vi "File - Load Controls from INI.vi"(7 "Section":string, 8 "error in (no error)":errorcluster, 9 "Array of References":refnum<vi>[](array[refnum]), 11 "INI File":path) -> (0 "error out":errorcluster)   [LabVIEW 2020]
doc: "Updates the values of controls (passed as an array of references) with the values read from an INI file.\n\nThe control names are used for the key names (with spaces removed).\n\nWorks with digital/boolean/string/path/VISAResourceName and single level clusters."
uses:
  <vilib>/Utility/config.llb/Read Key (Double).vi
  <vilib>/Utility/config.llb/Read Key (U32).vi
  <vilib>/Utility/config.llb/Read Key (String).vi
  <vilib>/Utility/config.llb/NI_LVConfig.lvlib
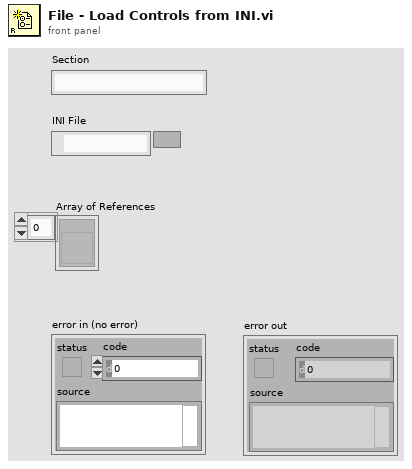
[diagram p1: front panel]
types:
  T1 = typedef "NI_LVConfig.lvlib/Config Data RefNum.ctl" = refnum<k1>
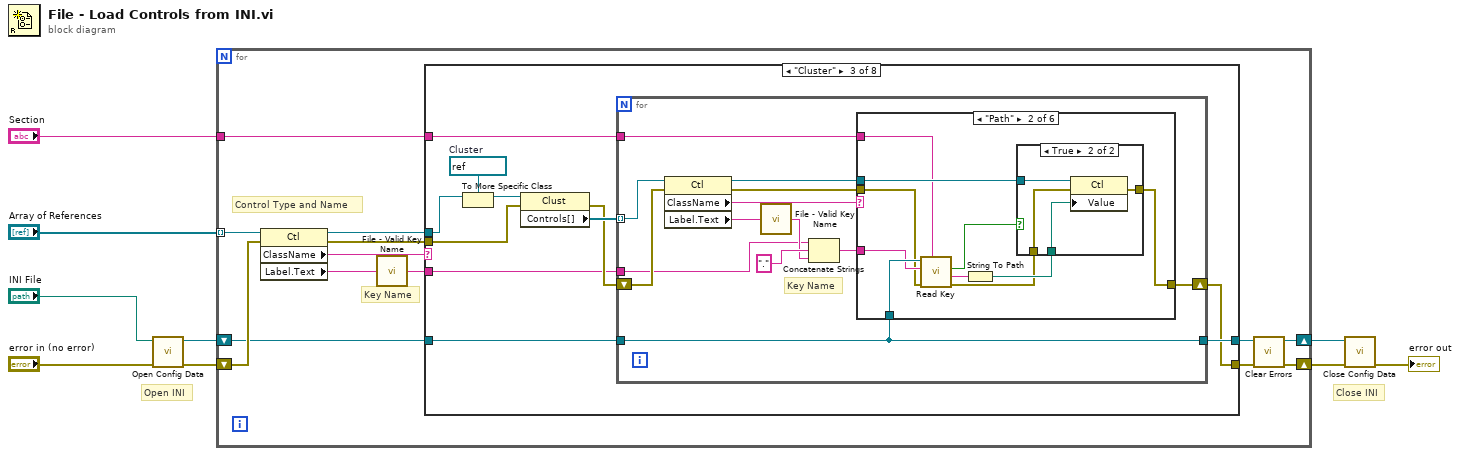
[diagram p0: block diagram]
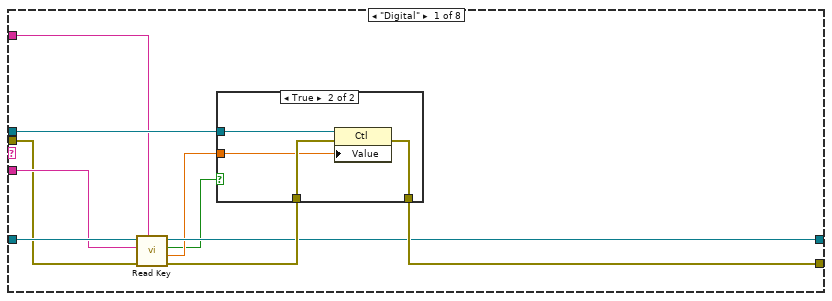
[diagram p2: hidden frame]
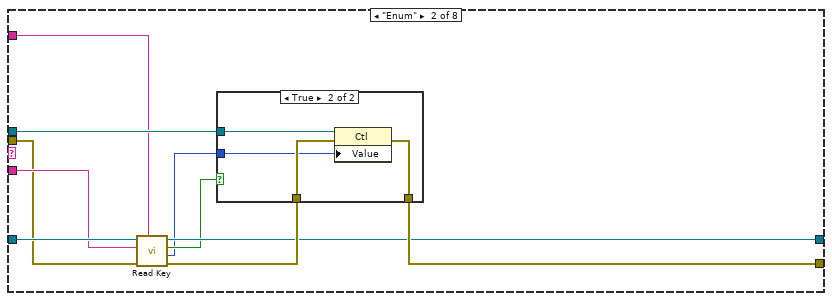
[diagram p4: hidden frame]
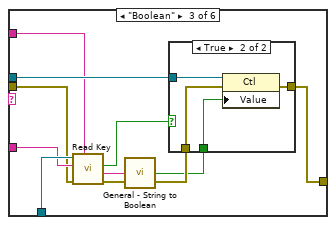
[diagram p8: hidden frame]
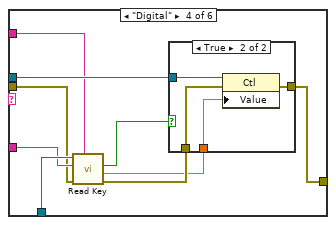
[diagram p10: hidden frame]
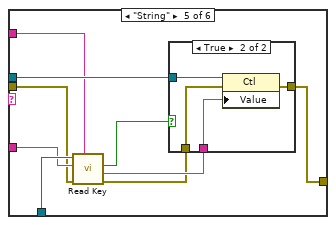
[diagram p12: hidden frame]
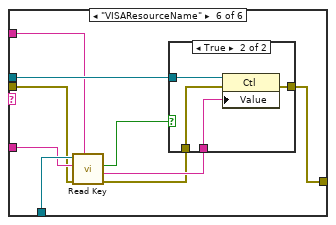
[diagram p14: hidden frame]
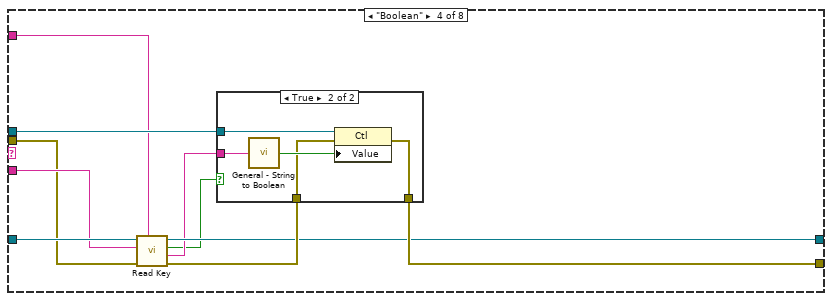
[diagram p16: hidden frame]
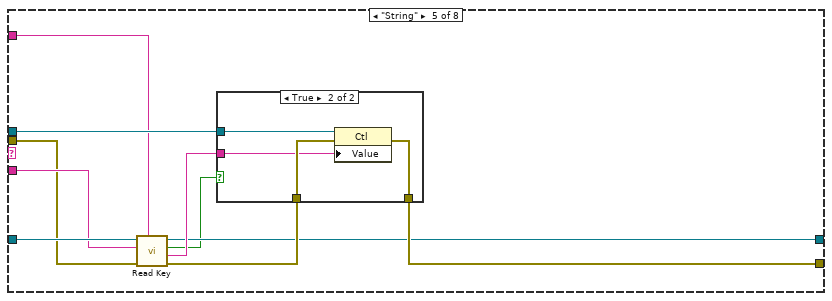
[diagram p18: hidden frame]
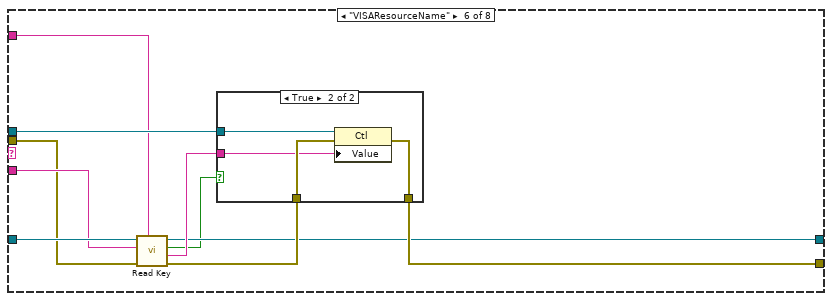
[diagram p20: hidden frame]
diagram:
  # "Close INI"
  # "Open INI"
  n1 = call <vilib>:"Open Config Data.vi"("error in (no error)"="error in (no error)", "configuration file path"="INI File") -> ("error out"=w6:errorcluster, "refnum"=w5:T1)  [unwired: 7 in, 1 out]
  n2 = for {
    tunnel: "Array of References" -> [w21] mode=indexing
    tunnel: "Section" -> [w18]
    shift-right: [w10] -> w3
    shift-left: w6 -> [w16]
    shift-right: [w14] -> w1
    shift-left: w5 -> [w15]
    # "Key Name"
    # "Control Type and Name"
    n3 = property class="Ctl"(reference=w21, error in=w16) -> (reference out=w19:refnum<vi>, error out=w11:errorcluster, "ClassName"=w20:string, "Label.Text"=w12:string)
    n4 = call "File - Valid Key Name.vi"("Key Name In"=w12) -> ("Key Name Out"=w13:string)  [unwired: 4 in]
    n5 = case shown="\"Cluster\"" w20 {
      tunnel: w19 -> [w31 w46 w60 w158 w174 w189 w204 _]
      tunnel: w13 -> [w23 w39 w54 w150 w166 w181 w196 _]
      tunnel: w18 -> [w26 w41 w53 w156 w171 w186 w200 _]
      tunnel: [w30 w45 w52 w157 w173 w188 w198 w211] -> w17
      tunnel: w15 -> [w28 w43 w59 w154 w169 w184 w202 w212]
      tunnel: [w27 w42 w58 w153 w168 w183 w203 w212] -> w14
      tunnel: w11 -> [w22 w38 w57 w149 w165 w180 w195 w211]
      frame "Digital" {
        n6 = call-poly <vilib>:"Read Key.vi"("section"=w26, "error in (no error)"=w22, "key"=w23, "refnum"=w28) -> ("error out"=w29:errorcluster, "value"=w25:dbl, "found?"=w24:bool, "refnum out"=w27:T1)  [unwired: 4 in]
        n7 = case shown="True" w24 {
          tunnel: w31 -> [_ w36]
          tunnel: [w32 w35] -> w30
          tunnel: w29 -> [w32 w34]
          tunnel: w25 -> [_ w33]
          frame False {
          }
          frame True {
            n8 = property class="Ctl"(reference=w36, error in=w34, "Value"=w33) -> (error out=w35:errorcluster)  [unwired: 1 out]
          }
        }
      }
      frame "Enum" {
        n9 = call-poly <vilib>:"Read Key.vi"("section"=w41, "error in (no error)"=w38, "key"=w39, "refnum"=w43) -> ("error out"=w44:errorcluster, "value"=w37:u32, "found?"=w40:bool, "refnum out"=w42:T1)  [unwired: 4 in]
        n10 = case shown="True" w40 {
          tunnel: w46 -> [_ w51]
          tunnel: [w47 w50] -> w45
          tunnel: w44 -> [w47 w49]
          tunnel: w37 -> [_ w48]
          frame False {
          }
          frame True {
            n11 = property class="Ctl"(reference=w51, error in=w49, "Value"=w48) -> (error out=w50:errorcluster)  [unwired: 1 out]
          }
        }
      }
      frame "Cluster" {
        w62 = refnum<vi> refnum  # Cluster
        n12 = To More Specific Class(target class=w62, reference=w60) -> (specific class reference=w61:refnum<vi>)  [unwired: 1 in, 1 out]
        n13 = property class="Clust"(reference=w61, error in=w57) -> (error out=w55:errorcluster, "Controls[]"=w56:refnum<vi>[])  [unwired: 1 out]
        n14 = for {
          tunnel: w59 -> [w66]
          tunnel: [w66] -> w58
          tunnel: w56 -> [w75] mode=indexing
          shift-right: [w63] -> w52
          shift-left: w55 -> [w74]
          tunnel: w54 -> [w70]
          tunnel: w53 -> [w65]
          # "Key Name"
          n15 = property class="Ctl"(reference=w75, error in=w74) -> (reference out=w69:refnum<vi>, error out=w64:errorcluster, "ClassName"=w67:string, "Label.Text"=w71:string)
          n16 = call "File - Valid Key Name.vi"("Key Name In"=w71) -> ("Key Name Out"=w72:string)  [unwired: 4 in]
          n17 = Concatenate Strings(w70, ".", w72) -> (w68:string)
          n18 = case shown="\"Path\"" w67 {
            tunnel: w69 -> [_ w86 w101 w115 w129 w143]
            tunnel: w68 -> [_ w81 w98 w112 w126 w140]
            tunnel: w66 -> [_ w85 w100 w114 w128 w142]
            tunnel: w65 -> [_ w80 w97 w111 w125 w139]
            tunnel: w64 -> [w76 w79 w96 w110 w124 w138]
            tunnel: [w76 w77 w94 w108 w121 w135] -> w63
            frame Default {
            }
            frame "Path" {
              n19 = call-poly <vilib>:"Read Key.vi"("section"=w80, "error in (no error)"=w79, "key"=w81, "refnum"=w85) -> ("error out"=w78:errorcluster, "value"=w83:string, "found?"=w82:bool)  [unwired: 4 in, 1 out]
              n20 = String To Path(string=w83) -> (path=w84:path)
              n21 = case shown="True" w82 {
                tunnel: w86 -> [_ w91]
                tunnel: w84 -> [_ w90]
                tunnel: [w87 w89] -> w77
                tunnel: w78 -> [w87 w88]
                frame False {
                }
                frame True {
                  n22 = property class="Ctl"(reference=w91, error in=w88, "Value"=w90) -> (error out=w89:errorcluster)  [unwired: 1 out]
                }
              }
            }
            frame "Boolean" {
              n23 = call-poly <vilib>:"Read Key.vi"("section"=w97, "error in (no error)"=w96, "key"=w98, "refnum"=w100) -> ("error out"=w95:errorcluster, "value"=w93:string, "found?"=w99:bool)  [unwired: 4 in, 1 out]
              n24 = call "General - String to Boolean.vi"("Text In"=w93) -> ("Boolean Out"=w92:bool)  [unwired: 4 in]
              n25 = case shown="True" w99 {
                tunnel: w101 -> [_ w106]
                tunnel: w92 -> [_ w105]
                tunnel: [w102 w104] -> w94
                tunnel: w95 -> [w102 w103]
                frame False {
                }
                frame True {
                  n26 = property class="Ctl"(reference=w106, error in=w103, "Value"=w105) -> (error out=w104:errorcluster)  [unwired: 1 out]
                }
              }
            }
            frame "Digital" {
              n27 = call-poly <vilib>:"Read Key.vi"("section"=w111, "error in (no error)"=w110, "key"=w112, "refnum"=w114) -> ("error out"=w109:errorcluster, "value"=w107:dbl, "found?"=w113:bool)  [unwired: 4 in, 1 out]
              n28 = case shown="True" w113 {
                tunnel: w115 -> [_ w120]
                tunnel: w107 -> [_ w119]
                tunnel: [w116 w118] -> w108
                tunnel: w109 -> [w116 w117]
                frame False {
                }
                frame True {
                  n29 = property class="Ctl"(reference=w120, error in=w117, "Value"=w119) -> (error out=w118:errorcluster)  [unwired: 1 out]
                }
              }
            }
            frame "String" {
              n30 = call-poly <vilib>:"Read Key.vi"("section"=w125, "error in (no error)"=w124, "key"=w126, "refnum"=w128) -> ("error out"=w122:errorcluster, "value"=w123:string, "found?"=w127:bool)  [unwired: 4 in, 1 out]
              n31 = case shown="True" w127 {
                tunnel: w129 -> [_ w134]
                tunnel: w123 -> [_ w133]
                tunnel: w122 -> [w130 w132]
                tunnel: [w130 w131] -> w121
                frame False {
                }
                frame True {
                  n32 = property class="Ctl"(reference=w134, error in=w132, "Value"=w133) -> (error out=w131:errorcluster)  [unwired: 1 out]
                }
              }
            }
            frame "VISAResourceName" {
              n33 = call-poly <vilib>:"Read Key.vi"("section"=w139, "error in (no error)"=w138, "key"=w140, "refnum"=w142) -> ("error out"=w136:errorcluster, "value"=w137:string, "found?"=w141:bool)  [unwired: 4 in, 1 out]
              n34 = case shown="True" w141 {
                tunnel: w143 -> [_ w148]
                tunnel: w137 -> [_ w147]
                tunnel: w136 -> [w144 w146]
                tunnel: [w144 w145] -> w135
                frame False {
                }
                frame True {
                  n35 = property class="Ctl"(reference=w148, error in=w146, "Value"=w147) -> (error out=w145:errorcluster)  [unwired: 1 out]
                }
              }
            }
          }
        }
      }
      frame "Boolean" {
        n36 = call-poly <vilib>:"Read Key.vi"("section"=w156, "error in (no error)"=w149, "key"=w150, "refnum"=w154) -> ("error out"=w155:errorcluster, "value"=w152:string, "found?"=w151:bool, "refnum out"=w153:T1)  [unwired: 4 in]
        n37 = case shown="True" w151 {
          tunnel: w158 -> [_ w164]
          tunnel: [w159 w162] -> w157
          tunnel: w155 -> [w159 w161]
          tunnel: w152 -> [_ w160]
          frame False {
          }
          frame True {
            n38 = call "General - String to Boolean.vi"("Text In"=w160) -> ("Boolean Out"=w163:bool)  [unwired: 4 in]
            n39 = property class="Ctl"(reference=w164, error in=w161, "Value"=w163) -> (error out=w162:errorcluster)  [unwired: 1 out]
          }
        }
      }
      frame "String" {
        n40 = call-poly <vilib>:"Read Key.vi"("section"=w171, "error in (no error)"=w165, "key"=w166, "refnum"=w169) -> ("error out"=w172:errorcluster, "value"=w170:string, "found?"=w167:bool, "refnum out"=w168:T1)  [unwired: 4 in]
        n41 = case shown="True" w167 {
          tunnel: w174 -> [_ w179]
          tunnel: [w175 w178] -> w173
          tunnel: w172 -> [w175 w177]
          tunnel: w170 -> [_ w176]
          frame False {
          }
          frame True {
            n42 = property class="Ctl"(reference=w179, error in=w177, "Value"=w176) -> (error out=w178:errorcluster)  [unwired: 1 out]
          }
        }
      }
      frame "VISAResourceName" {
        n43 = call-poly <vilib>:"Read Key.vi"("section"=w186, "error in (no error)"=w180, "key"=w181, "refnum"=w184) -> ("error out"=w187:errorcluster, "value"=w185:string, "found?"=w182:bool, "refnum out"=w183:T1)  [unwired: 4 in]
        n44 = case shown="True" w182 {
          tunnel: w189 -> [_ w194]
          tunnel: [w190 w193] -> w188
          tunnel: w187 -> [w190 w192]
          tunnel: w185 -> [_ w191]
          frame False {
          }
          frame True {
            n45 = property class="Ctl"(reference=w194, error in=w192, "Value"=w191) -> (error out=w193:errorcluster)  [unwired: 1 out]
          }
        }
      }
      frame "Path" {
        n46 = call-poly <vilib>:"Read Key.vi"("section"=w200, "error in (no error)"=w195, "key"=w196, "refnum"=w202) -> ("error out"=w199:errorcluster, "value"=w201:string, "found?"=w197:bool, "refnum out"=w203:T1)  [unwired: 4 in]
        n47 = case shown="True" w197 {
          tunnel: w204 -> [_ w210]
          tunnel: w201 -> [_ w208]
          tunnel: w199 -> [w205 w207]
          tunnel: [w205 w206] -> w198
          frame False {
          }
          frame True {
            n48 = String To Path(string=w208) -> (path=w209:path)
            n49 = property class="Ctl"(reference=w210, error in=w207, "Value"=w209) -> (error out=w206:errorcluster)  [unwired: 1 out]
          }
        }
      }
      frame Default {
      }
    }
    n50 = call <vilib>:"Clear Errors.vi"("error in (no error)"=w17) -> ("error out"=w10:errorcluster)  [unwired: 5 in, 1 out]
  }
  n51 = call <vilib>:"Close Config Data.vi"("error in (no error)"=w3, "refnum"=w1) -> ("error out"=→"error out":errorcluster)  [unwired: 8 in, 1 out]
